vi "Set Sessions.vi"(11 "Semiconductor Module Context":T1) -> (0 "error out":errorcluster)   [LabVIEW 2013]
uses:
  <vilib>/NI_TestStand_SemiconductorModule/NI_TestStand_Semiconductor_Module.lvlibp/PinMap/General/SemiconductorModuleContext.ctl
  <vilib>/NI_TestStand_SemiconductorModule/NI_TestStand_Semiconductor_Module.lvlibp
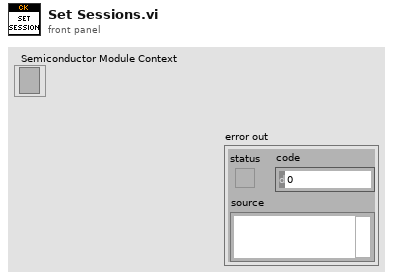
[diagram p1: front panel]
types:
  T1 = typedef "NI_TestStand_Semiconductor_Module.lvlibp/SemiconductorModuleContext.ctl" = refnum<k7>
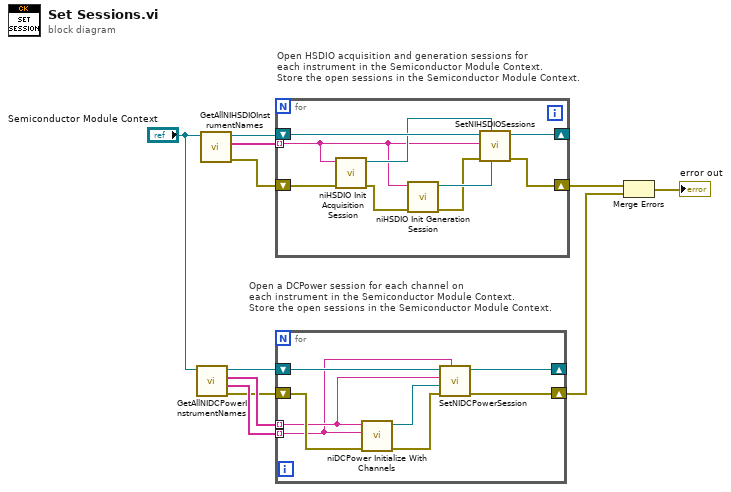
[diagram p0: block diagram]
diagram:
  # "Open a DCPower session for each channel on \neach instrument in the Semiconductor Module Context.\nStore the open sessions in the Semiconductor Module Context."
  # "Open HSDIO acquisition and generation sessions for\neach instrument in the Semiconductor Module Context.\nStore the open sessions in the Semiconductor Module Context."
  n1 = call <vilib>:"GetAllNIDCPowerInstrumentNames.vi"("Semiconductor Module Context"="Semiconductor Module Context") -> ("error out"=w4:errorcluster, "Channel Ids"=w5:string[], "Instrument Names"=w10:string[], "Semiconductor Module Context Out"=w9:T1)  [unwired: 7 in]
  n2 = call <vilib>:"GetAllNIHSDIOInstrumentNames.vi"("Semiconductor Module Context"="Semiconductor Module Context") -> ("error out"=w2:errorcluster, "Instrument Names"=w11:string[], "Semiconductor Module Context Out"=w3:T1)  [unwired: 8 in]
  n3 = for {
    tunnel: w11 -> [w13] mode=indexing
    shift-right: [w15] -> w8
    shift-left: w2 -> [w20]
    shift-right: [w17] -> _
    shift-left: w3 -> [w19]
    n4 = call <instrlib>:"niHSDIO Init Acquisition Session.vi"("error in (no error)"=w20, "resource name"=w13) -> ("error out"=w14:errorcluster, "instrument handle out"=w18:refnum<k15>)  [unwired: 8 in]
    n5 = call <instrlib>:"niHSDIO Init Generation Session.vi"("error in (no error)"=w14, "resource name"=w13) -> ("error out"=w12:errorcluster, "instrument handle out"=w16:refnum<k15>)  [unwired: 8 in]
    n6 = call <vilib>:"SetNIHSDIOSessions.vi"("Generation Session"=w16, "Acquisition Session"=w18, "error in (no error)"=w12, "Instrument Name"=w13, "Semiconductor Module Context"=w19) -> ("error out"=w15:errorcluster, "Semiconductor Module Context Out"=w17:T1)  [unwired: 5 in]
  }
  n7 = for {
    tunnel: w10 -> [w24] mode=indexing
    shift-right: [w27] -> _
    shift-left: w9 -> [w28]
    shift-right: [w26] -> w7
    shift-left: w4 -> [w25]
    tunnel: w5 -> [w21] mode=indexing
    n8 = call <instrlib>:"niDCPower Initialize With Channels.vi"("error in (no error)"=w25, "channels"=w21, "resource name"=w24) -> ("error out"=w23:errorcluster, "instrument handle out"=w22:refnum<k15>)  [unwired: 7 in]
    n9 = call <vilib>:"SetNIDCPowerSession.vi"("Channel Id"=w21, "error in (no error)"=w23, "Instrument Session"=w22, "Instrument Name"=w24, "Semiconductor Module Context"=w28) -> ("error out"=w26:errorcluster, "Semiconductor Module Context Out"=w27:T1)  [unwired: 5 in]
  }
  n10 = Merge Errors(w8, w7) -> (→"error out":errorcluster)
